vi "niRFUtil MT UTIL Perform Resampling.vi"   [LabVIEW 2015, in "niRFUtil.lvlib"]
uses:
  niRFUtil.lvlib
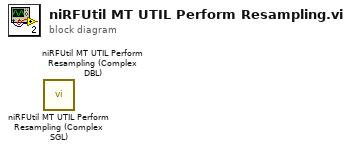
[diagram p0: block diagram]
diagram:
  n1 = call "niRFUtil MT UTIL Perform Resampling (Complex SGL).vi"() -> ()  [unwired: 13 in, 3 out]
  n2 = call "niRFUtil MT UTIL Perform Resampling (Complex DBL).vi"() -> ()  [unwired: 13 in, 3 out]
